vi "标准偏差.vi"() -> ()   [LabVIEW 2018]
uses:
  <vilib>/Analysis/1siggen.llb/General Gauss-Mod Sine.vi
  <vilib>/Analysis/NI_AALBase.lvlib
panel:
  out "variance":dbl caption="方差" format="%0.2f"
  out "standard deviation":dbl caption="标准差" format="%0.2f"
  out "mean":dbl caption="均值" format="%0.2f"
  in  "停止":bool
  in  "Weighting (Sample)":enum16{"Sample", "Population"}(ring) caption="权（采样）"
  out "波形图":dbl[](graph)
  in  "波形类型":bool
  in  "频率":dbl
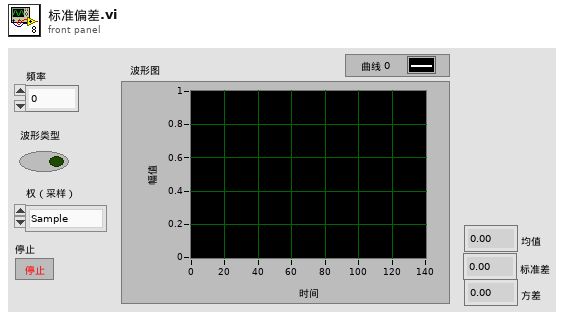
[diagram p1: front panel]
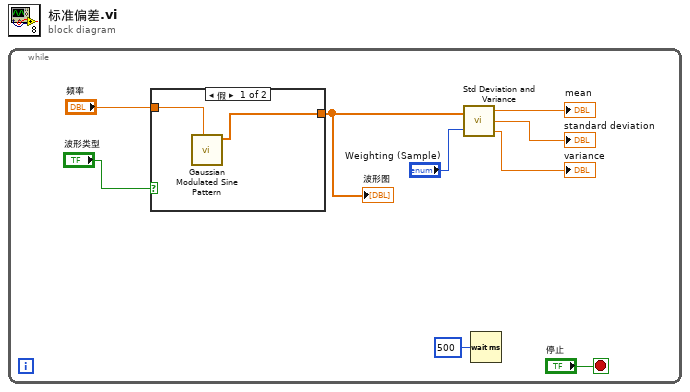
[diagram p0: block diagram]
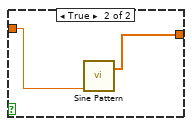
[diagram p2: hidden frame]
diagram:
  n1 = while {
    stop <- "停止" stop-if-true
    n2 = case shown="假" "波形类型" {
      tunnel: "频率" -> [w11 w13]
      tunnel: [w10 w12] -> w6
      frame False {
        n3 = call <vilib>:"Gaussian Modulated Sine Pattern.vi"("center frequency (Hz)"=w11) -> ("Gauss-Mod Sine Pattern"=w10:dbl[])  [unwired: 9 in, 1 out]
      }
      frame True {
        n4 = call <vilib>:"Sine Pattern.vi"("cycles"=w13) -> ("Sinusoidal Pattern"=w12:dbl[])  [unwired: 3 in, 1 out]
      }
    }
    "波形图" <- w6
    n5 = call <vilib>:"Std Deviation and Variance.vi"("X"=w6, "Weighting (Sample)"="Weighting (Sample)") -> ("mean"=→"mean":dbl, "standard deviation"=→"standard deviation":dbl, "variance"=→"variance":dbl)
    n6 = Wait (ms)(milliseconds to wait=u32 500 ("等待时间（毫秒）")) -> ()  [unwired: 1 out]
  }
